vi "Get Active Assert Name.vi"(9 "Coords":T1, 11 "CtlRef":refnum<vi>) -> (0 "error out":errorcluster, 2 "Active Assert Name":string)   [LabVIEW 2016, in "Assert API Components.lvlib" / "Assert Display.lvlib" / "Main Display.lvlib" / "Main Display.lvclass"]
doc: "Gets the name of an assert based on the cursor position within the listbox control"
uses:
  Main Display.lvclass
  <vilib>/Utility/miscctls.llb/LVPoint32TypeDef.ctl
  <resource>/AFDebug/Localized Strings.vi
  <resource>/AFDebug/Get Clone Name.vi
  <resource>/AFDebug/Actor Registry.vi
  <resource>/AFDebug/TDM Registry.vi
  <resource>/AFDebug/AF Debug.lvlib
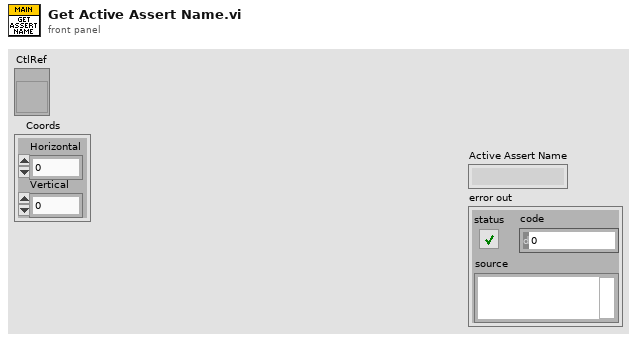
[diagram p1: front panel]
types:
  T1 = typedef "LVPoint32TypeDef.ctl" = cluster{"Horizontal":i32, "Vertical":i32}
  T2 = typedef "LVRowAndColumnTypeDef.ctl" = cluster{"Row":i32, "Column":i32}
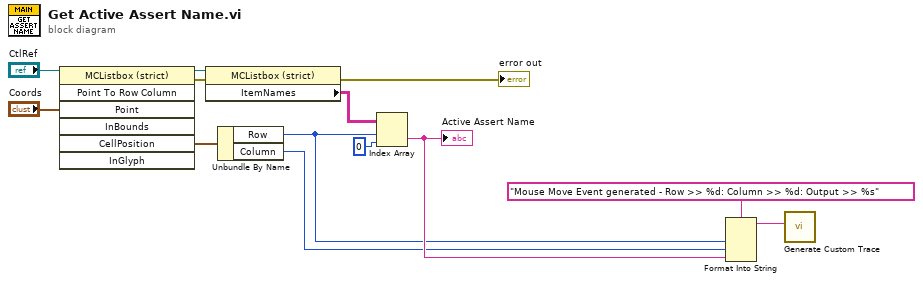
[diagram p0: block diagram]
diagram:
  n1 = invoke class="MCListbox (strict)" method="Point To Row Column"(reference="CtlRef", "Point"="Coords") -> (reference out=w10:refnum<vi>, error out=w9:errorcluster, "CellPosition"=w11:T2)  [unwired: 5 in, 4 out]
  n2 = property class="MCListbox (strict)"(reference=w10, error in=w9) -> (error out=→"error out":errorcluster, "ItemNames"=w8:string[][])  [unwired: 1 out]
  n3 = Unbundle By Name(w11) -> ("Row"=w3:i32, "Column"=w4:i32)
  n4 = Index Array(array=w8, index (row)=w3, index (col)=0 ("disabled index (col)")) -> (element=w5:string)
  "Active Assert Name" <- w5
  n5 = Format Into String(format string="Mouse Move Event generated - Row >> %d: Column >> %d: Output >> %s", w3, w4, w5) -> (resulting string=w2:string)  [unwired: 2 in, 1 out]
  n6 = call <resource>:"Generate Custom Trace.vi"("Custom Action"=w2) -> ()  [unwired: 11 in]
